vi "阈值设定.vi"() -> ()   [LabVIEW 2014]
uses:
  <vilib>/vision/Image Controls.llb/IMAQ Image.ctl
  <vilib>/Utility/error.llb/DialogType.ctl
  <vilib>/Utility/file.llb/Write To Spreadsheet File (I64).vi
  <vilib>/vision/NI_Vision_Development_Module.lvlib
panel:
  out "?":T1(plugin-control)
  in  "刷新按钮":bool
  in  "停止运算":bool
  in  "下一步":bool
  out "Histogram 3":dynamicdata(graph) caption="B直方图"
  out "Histogram 2":dynamicdata(graph) caption="A直方图"
  out "Histogram":dynamicdata(graph) caption="L直方图"
  in  "b颜色通道":cluster{i32, i32}(slide)={-21, 6} scale=-100.0..100.0
  in  "a颜色通道":cluster{i32, i32}(slide)={-21, -7} scale=-100.0..100.0
  in  "L颜色通道":cluster{i32, i32}(slide)={81, 99} scale=0.0..100.0
  out "lie":i32
  out "hang":i32
  out "颜色空间处理后的图，提取火焰":T1(plugin-control)
  in  "Image 4":T1
  out "B":u8[][](array[numeric])
  out "G":u8[][](array[numeric])
  out "R":u8[][](array[numeric])
  out "原图":T1(plugin-control)
  # "Lab颜色空间阈值选择"
  # "Lab颜色分割图像"
  # "滤波平滑图像"
  # "原图"
  # "阈\n值\n选\n择"
  # "火\n焰\n颜\n色\n直\n方\n图"
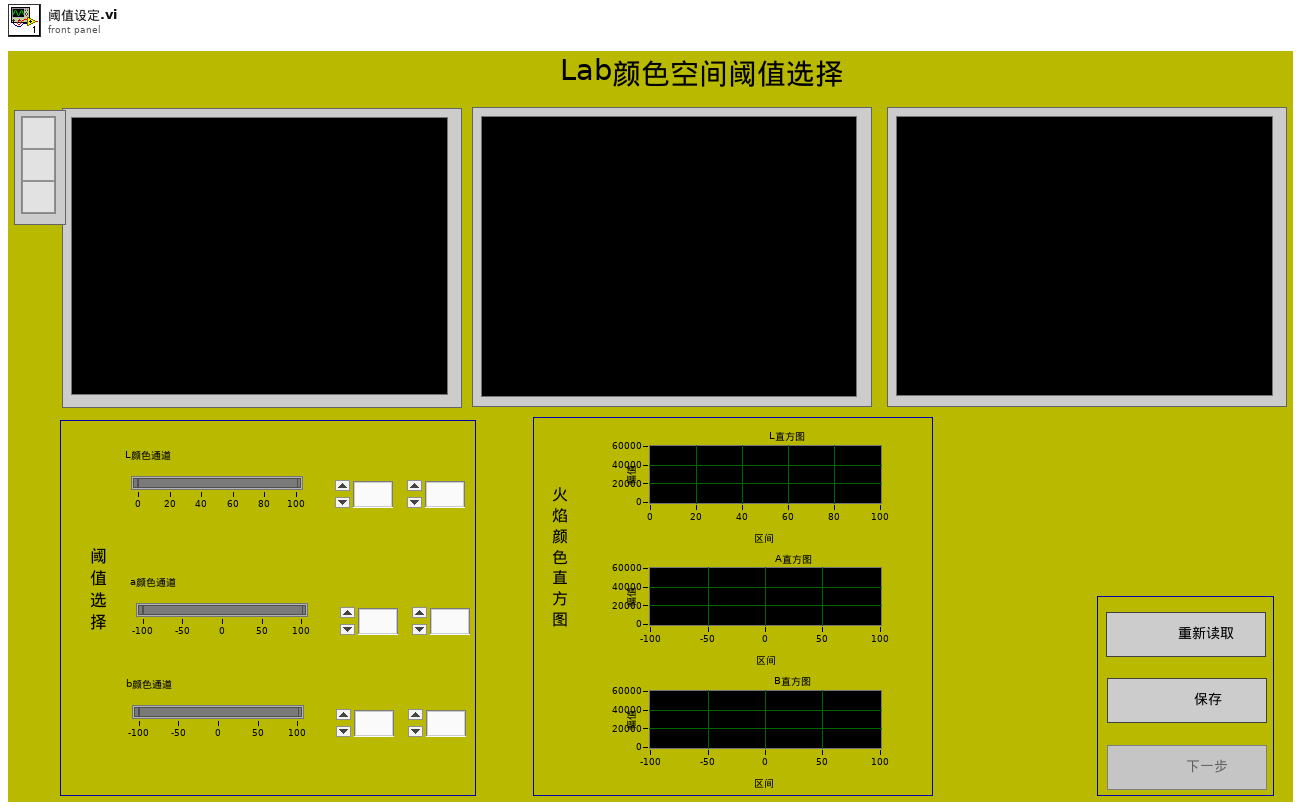
[diagram p1: front panel]
types:
  T1 = typedef "IMAQ Image.ctl" = refnum<image>
  T2 = enum8{"Enabled", "Disabled", "Disabled and Grayed Out"}
  T3 = enum32{"Invalid", "Standard", "Closed", "Hidden", "Minimized", "Maximized"}
  T4 = typedef "Image Type" = u32
  T5 = typedef "DialogType.ctl" = u16
  T6 = cluster{"Global Rectangle":i32[], "Contours":cluster{"Contour Type":u32, "ROI Type":u32, "Points":i32[]}[]}
  T7 = typedef "IMAQ Rectangle" = cluster{"Left":i32, "Top":i32, "Right":i32, "Bottom":i32, "Rotation":dbl}
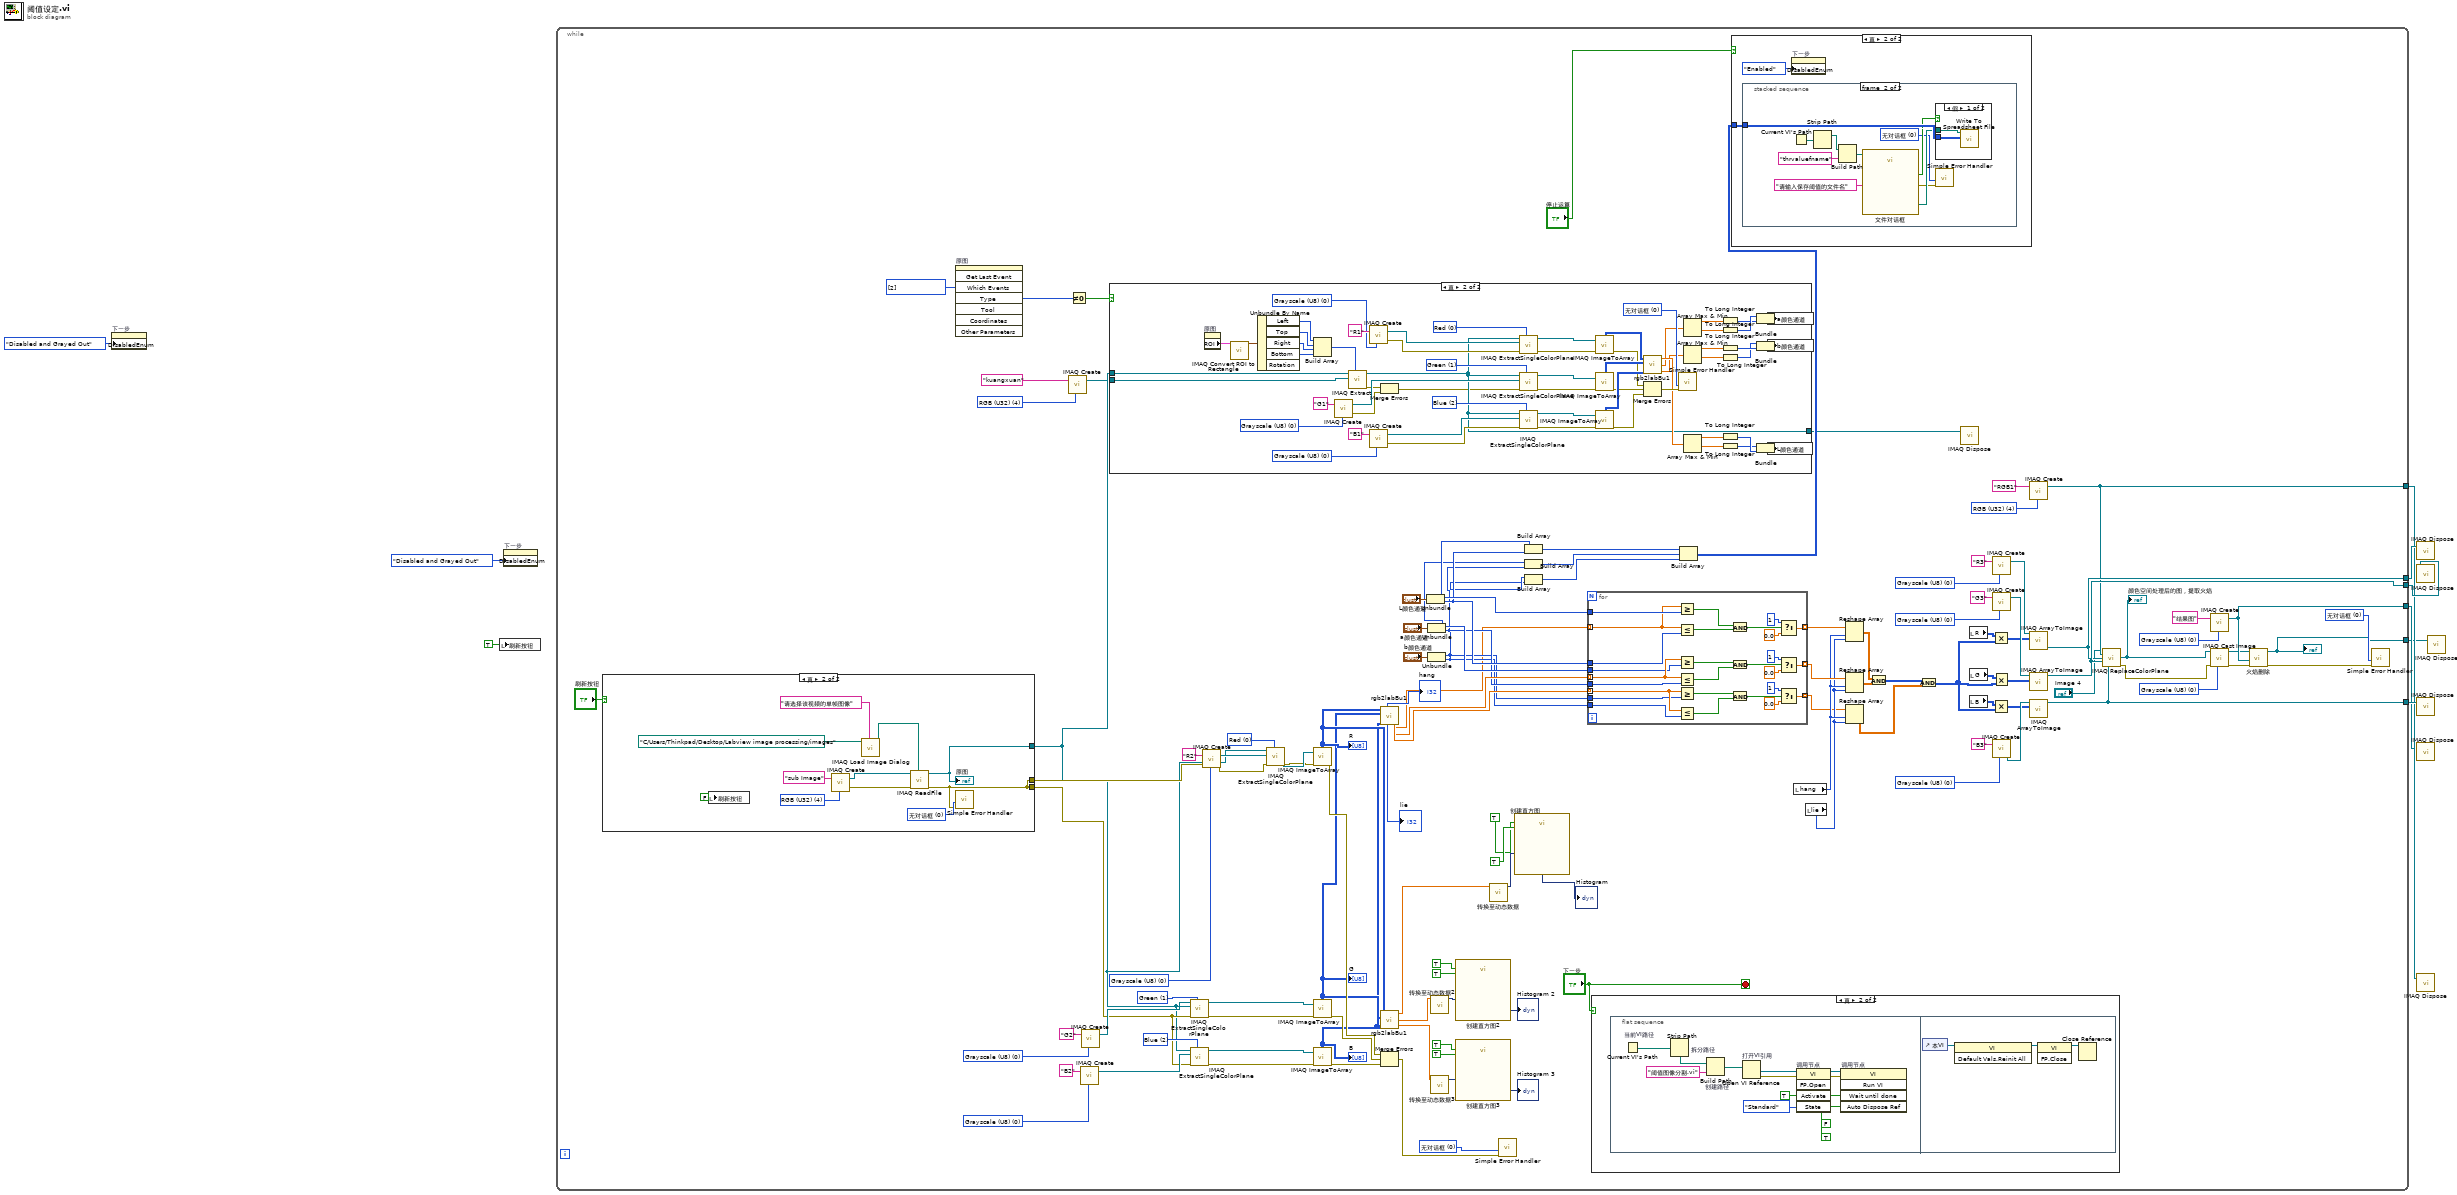
[diagram p0: block diagram]
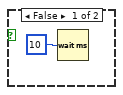
[diagram p2: hidden frame]
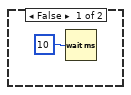
[diagram p3: hidden frame]
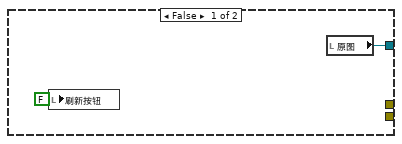
[diagram p4: hidden frame]
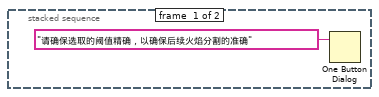
[diagram p6: hidden frame]
diagram:
  n1 = property on="下一步" class="Bool"("DisabledEnum"=T2."Disabled and Grayed Out" ("禁用")) -> ()  [unwired: 2 in, 2 out]
  n2 = local write "刷新按钮"(TRUE ("布尔")) -> ()
  n3 = property on="下一步" class="Bool"("DisabledEnum"=T2."Disabled and Grayed Out" ("禁用")) -> ()  [unwired: 2 in, 2 out]
  n4 = while {
    tunnel: [w125] -> w8
    tunnel: [w124] -> w7
    tunnel: [w123] -> w6
    tunnel: [w122] -> w5
    tunnel: [w121] -> w4
    tunnel: [w10] -> w1
    stop <- "下一步" stop-if-true
    w16 = T4 4 items=["Grayscale (U8)", "Grayscale (I16)", "Grayscale (SGL)", "Complex (CSG)", "RGB (U32)", "HSL (U32)", "RGB (U64)", "Grayscale (U16)"] ("Image Type")
    w15 = i32[] [2] items=["No  event", "Click event", "Draw event", "Move event", "Size event", "Scroll event", "Activate event", "Close event", "Double click event"] ("Events list (all)")
    w29 = T4 0 items=["Grayscale (U8)", "Grayscale (I16)", "Grayscale (SGL)", "Complex (CSG)", "RGB (U32)", "HSL (U32)", "RGB (U64)", "Grayscale (U16)"] ("Image Type")
    w27 = T4 0 items=["Grayscale (U8)", "Grayscale (I16)", "Grayscale (SGL)", "Complex (CSG)", "RGB (U32)", "HSL (U32)", "RGB (U64)", "Grayscale (U16)"] ("Image Type")
    w25 = T4 0 items=["Grayscale (U8)", "Grayscale (I16)", "Grayscale (SGL)", "Complex (CSG)", "RGB (U32)", "HSL (U32)", "RGB (U64)", "Grayscale (U16)"] ("Image Type")
    w56 = T5 0 items=["无对话框", "确定信息", "继续或停止信息", "确定信息＋警告", "继续/停止+警告"] ("type of dialog (OK msg:1)")
    w78 = T4 0 items=["Grayscale (U8)", "Grayscale (I16)", "Grayscale (SGL)", "Complex (CSG)", "RGB (U32)", "HSL (U32)", "RGB (U64)", "Grayscale (U16)"] ("Image Type")
    w79 = T4 4 items=["Grayscale (U8)", "Grayscale (I16)", "Grayscale (SGL)", "Complex (CSG)", "RGB (U32)", "HSL (U32)", "RGB (U64)", "Grayscale (U16)"] ("Image Type")
    w94 = T4 0 items=["Grayscale (U8)", "Grayscale (I16)", "Grayscale (SGL)", "Complex (CSG)", "RGB (U32)", "HSL (U32)", "RGB (U64)", "Grayscale (U16)"] ("Image Type")
    w100 = T4 0 items=["Grayscale (U8)", "Grayscale (I16)", "Grayscale (SGL)", "Complex (CSG)", "RGB (U32)", "HSL (U32)", "RGB (U64)", "Grayscale (U16)"] ("Image Type")
    w98 = T4 0 items=["Grayscale (U8)", "Grayscale (I16)", "Grayscale (SGL)", "Complex (CSG)", "RGB (U32)", "HSL (U32)", "RGB (U64)", "Grayscale (U16)"] ("Image Type")
    w103 = T4 0 items=["Grayscale (U8)", "Grayscale (I16)", "Grayscale (SGL)", "Complex (CSG)", "RGB (U32)", "HSL (U32)", "RGB (U64)", "Grayscale (U16)"] ("Image Type")
    w105 = T5 0 items=["无对话框", "确定信息", "继续或停止信息", "确定信息＋警告", "继续/停止+警告"] ("type of dialog (OK msg:1)")
    w114 = 2 items=["Red", "Green", "Blue", "Hue", "Saturation", "Luminance", "Value", "Intensity"] ("Color Plane")
    w115 = 1 items=["Red", "Green", "Blue", "Hue", "Saturation", "Luminance", "Value", "Intensity"] ("Color Plane")
    w116 = 0 items=["Red", "Green", "Blue", "Hue", "Saturation", "Luminance", "Value", "Intensity"] ("Color Plane")
    n5 = case shown="真" "刷新按钮" {
      tunnel: [_ w205] -> w20
      tunnel: [w203 w206] -> w19
      tunnel: [_ w205] -> w32
      frame False {
        n6 = local write "刷新按钮"(FALSE ("布尔")) -> ()
        n7 = local read "原图"() -> (w203:T1)
      }
      frame True {
        w210 = T5 0 items=["无对话框", "确定信息", "继续或停止信息", "确定信息＋警告", "继续/停止+警告"] ("type of dialog (OK msg:1)")
        w213 = T4 4 items=["Grayscale (U8)", "Grayscale (I16)", "Grayscale (SGL)", "Complex (CSG)", "RGB (U32)", "HSL (U32)", "RGB (U64)", "Grayscale (U16)"] ("Image Type")
        n8 = local write "刷新按钮"(FALSE ("布尔")) -> ()
        n9 = call "IMAQ Create"("Image Name"="sub Image", "Image Type"=w213) -> ("New Image"=w212:T1, "error out"=w211:errorcluster)  [unwired: 2 in, 1 out]
        n10 = call "IMAQ Load Image Dialog"("Prompt"="请选择该视频的单帧图像", "Start Path"=path "C:/Users/Thinkpad/Desktop/Labview image processing/images") -> ("Path"=w207:path)  [unwired: 7 in, 2 out]
        n11 = call "IMAQ ReadFile"("File Path"=w207, "error in (no error)"=w211, "Image"=w212) -> ("error out"=w205:errorcluster, "Image Out"=w206:T1)  [unwired: 4 in, 3 out]
        "原图" <- w206
        n12 = call <vilib>:"Simple Error Handler.vi"("type of dialog (OK msg:1)"=w210, "error in (no error)"=w205) -> ()  [unwired: 3 in, 5 out]
      }
    }
    n13 = invoke on="原图" class="ImageControl" method="Get Last Event"("Which Events"=w15) -> ("Type"=w14:i32)  [unwired: 7 in, 7 out]
    n14 = call "IMAQ Create"("Image Name"="kuangxuan", "Image Type"=w16) -> ("New Image"=w18:T1)  [unwired: 2 in, 2 out]
    n15 = Not Equal To 0?(x=w14) -> (x != 0?=w13:bool)
    n16 = call "IMAQ Create"("Image Name"="B2", "Image Type"=w29) -> ("New Image"=w24:T1)  [unwired: 2 in, 2 out]
    n17 = call "IMAQ Create"("Image Name"="G2", "Image Type"=w27) -> ("New Image"=w23:T1)  [unwired: 2 in, 2 out]
    n18 = case shown="真" w13 {
      tunnel: w18 -> [_ w148]
      tunnel: [_ w147] -> w12
      tunnel: w19 -> [_ w146]
      frame False {
        n19 = Wait (ms)(milliseconds to wait=u32 10) -> ()  [unwired: 1 out]
      }
      frame True {
        w178 = T5 0 items=["无对话框", "确定信息", "继续或停止信息", "确定信息＋警告", "继续/停止+警告"] ("type of dialog (OK msg:1)")
        w189 = 2 items=["Red", "Green", "Blue", "Hue", "Saturation", "Luminance", "Value", "Intensity"] ("Color Plane")
        w190 = 1 items=["Red", "Green", "Blue", "Hue", "Saturation", "Luminance", "Value", "Intensity"] ("Color Plane")
        w191 = 0 items=["Red", "Green", "Blue", "Hue", "Saturation", "Luminance", "Value", "Intensity"] ("Color Plane")
        w195 = T4 0 items=["Grayscale (U8)", "Grayscale (I16)", "Grayscale (SGL)", "Complex (CSG)", "RGB (U32)", "HSL (U32)", "RGB (U64)", "Grayscale (U16)"] ("Image Type")
        w197 = T4 0 items=["Grayscale (U8)", "Grayscale (I16)", "Grayscale (SGL)", "Complex (CSG)", "RGB (U32)", "HSL (U32)", "RGB (U64)", "Grayscale (U16)"] ("Image Type")
        w199 = T4 0 items=["Grayscale (U8)", "Grayscale (I16)", "Grayscale (SGL)", "Complex (CSG)", "RGB (U32)", "HSL (U32)", "RGB (U64)", "Grayscale (U16)"] ("Image Type")
        n20 = property on="原图" class="ImageControl"() -> ("ROI"=w149:T6)  [unwired: 2 in, 2 out]
        n21 = call "IMAQ Convert ROI to Rectangle"("ROI Descriptor"=w149) -> ("Rectangle"=w155:T7)  [unwired: 8 in, 1 out]
        n22 = Unbundle By Name(w155) -> ("Left"=w154:i32, "Top"=w153:i32, "Right"=w152:i32, "Bottom"=w151:i32)  [unwired: 1 out]
        n23 = Build Array(w154, w153, w152, w151) -> (w150:i32[])
        n24 = call "IMAQ Create"("Image Name"="G1", "Image Type"=w197) -> ("New Image"=w193:T1, "error out"=w144:errorcluster)  [unwired: 2 in, 1 out]
        n25 = call "IMAQ Extract"("Optional Rectangle"=w150, "Image Dst"=w148, "Image Src"=w146) -> ("error out"=w145:errorcluster, "Image Dst Out"=w147:T1)  [unwired: 7 in]
        n26 = call "IMAQ Create"("Image Name"="R1", "Image Type"=w199) -> ("New Image"=w194:T1, "error out"=w184:errorcluster)  [unwired: 2 in, 1 out]
        n27 = call "IMAQ Create"("Image Name"="B1", "Image Type"=w195) -> ("New Image"=w192:T1, "error out"=w201:errorcluster)  [unwired: 2 in, 1 out]
        n28 = Merge Errors(w145, w144) -> (w143:errorcluster)
        n29 = call "IMAQ ExtractSingleColorPlane"("Color Plane"=w191, "error in (no error)"=w184, "Image Dst"=w194, "Image Src"=w147) -> ("error out"=w183:errorcluster, "Image Dst Out"=w158:T1)  [unwired: 6 in]
        n30 = call "IMAQ ExtractSingleColorPlane"("Color Plane"=w190, "error in (no error)"=w143, "Image Dst"=w193, "Image Src"=w147) -> ("error out"=w185:errorcluster, "Image Dst Out"=w157:T1)  [unwired: 6 in]
        n31 = call "IMAQ ExtractSingleColorPlane"("Color Plane"=w189, "error in (no error)"=w201, "Image Dst"=w192, "Image Src"=w147) -> ("error out"=w182:errorcluster, "Image Dst Out"=w156:T1)  [unwired: 6 in]
        n32 = call "IMAQ ImageToArray"("error in (no error)"=w183, "Image"=w158) -> ("error out"=w181:errorcluster, "Image Pixels (U8)"=w188:u8[][])  [unwired: 2 in, 3 out]
        n33 = call "IMAQ ImageToArray"("error in (no error)"=w185, "Image"=w157) -> ("error out"=w180:errorcluster, "Image Pixels (U8)"=w187:u8[][])  [unwired: 2 in, 3 out]
        n34 = call "IMAQ ImageToArray"("error in (no error)"=w182, "Image"=w156) -> ("error out"=w179:errorcluster, "Image Pixels (U8)"=w186:u8[][])  [unwired: 2 in, 3 out]
        n35 = call "rgb2labBu1.vi"("R"=w188, "G"=w187, "B"=w186) -> ("LZ"=w171:dbl[], "aZ"=w160:dbl[], "bZ"=w159:dbl[])  [unwired: 1 in, 2 out]
        n36 = Merge Errors(w181, w180, w179) -> (w177:errorcluster)
        n37 = call <vilib>:"Simple Error Handler.vi"("type of dialog (OK msg:1)"=w178, "error in (no error)"=w177) -> ()  [unwired: 3 in, 5 out]
        n38 = Array Max & Min(array=w160) -> (max value=w166:dbl, min value=w167:dbl)  [unwired: 2 out]
        n39 = Array Max & Min(array=w159) -> (max value=w165:dbl, min value=w164:dbl)  [unwired: 2 out]
        n40 = Array Max & Min(array=w171) -> (max value=w176:dbl, min value=w175:dbl)  [unwired: 2 out]
        n41 = To Long Integer(number=w166) -> (32bit integer=w169:i32)
        n42 = To Long Integer(number=w167) -> (32bit integer=w170:i32)
        n43 = To Long Integer(number=w165) -> (32bit integer=w162:i32)
        n44 = To Long Integer(number=w164) -> (32bit integer=w161:i32)
        n45 = To Long Integer(number=w176) -> (32bit integer=w173:i32)
        n46 = To Long Integer(number=w175) -> (32bit integer=w172:i32)
        n47 = Bundle(w170, w169) -> (w168:cluster{i32, i32})  [unwired: 1 in]
        n48 = Bundle(w161, w162) -> (w163:cluster{i32, i32})  [unwired: 1 in]
        n49 = Bundle(w172, w173) -> (w174:cluster{i32, i32})  [unwired: 1 in]
        n50 = local write "a颜色通道"(w168) -> ()
        n51 = local write "b颜色通道"(w163) -> ()
        n52 = local write "L颜色通道"(w174) -> ()
      }
    }
    n53 = call "IMAQ ExtractSingleColorPlane"("Color Plane"=w115, "error in (no error)"=w20, "Image Dst"=w23, "Image Src"=w19) -> ("error out"=w111:errorcluster, "Image Dst Out"=w119:T1)  [unwired: 6 in]
    n54 = call "IMAQ ExtractSingleColorPlane"("Color Plane"=w114, "error in (no error)"=w20, "Image Dst"=w24, "Image Src"=w19) -> ("error out"=w109:errorcluster, "Image Dst Out"=w54:T1)  [unwired: 6 in]
    n55 = call "IMAQ Create"("Image Name"="R2", "Image Type"=w25, "error in (no error)"=w32) -> ("New Image"=w22:T1, "error out"=w21:errorcluster)  [unwired: 1 in, 1 out]
    n56 = call "IMAQ ExtractSingleColorPlane"("Color Plane"=w116, "error in (no error)"=w21, "Image Dst"=w22, "Image Src"=w19) -> ("error out"=w110:errorcluster, "Image Dst Out"=w120:T1)  [unwired: 6 in]
    n57 = call "IMAQ ImageToArray"("error in (no error)"=w110, "Image"=w120) -> ("error out"=w108:errorcluster, "Image Pixels (U8)"=w42:u8[][])  [unwired: 2 in, 3 out]
    "R" <- w42
    n58 = call "IMAQ ImageToArray"("error in (no error)"=w111, "Image"=w119) -> ("error out"=w107:errorcluster, "Image Pixels (U8)"=w41:u8[][])  [unwired: 2 in, 3 out]
    "G" <- w41
    n59 = call "IMAQ ImageToArray"("error in (no error)"=w109, "Image"=w54) -> ("error out"=w106:errorcluster, "Image Pixels (U8)"=w40:u8[][])  [unwired: 2 in, 3 out]
    "B" <- w40
    n60 = call "rgb2labBu1.vi"("R"=w42, "G"=w41, "B"=w40) -> ("hang"=→"hang":i32, "lie"=→"lie":i32, "LZ"=w53:dbl[], "aZ"=w117:dbl[], "bZ"=w118:dbl[])  [unwired: 1 in]
    n61 = call "rgb2labBu1.vi"("R"=w42, "G"=w41, "B"=w40) -> ("LZ"=w39:dbl[], "aZ"=w44:dbl[], "bZ"=w48:dbl[])  [unwired: 1 in, 2 out]
    n62 = Merge Errors(w108, w107, w106) -> (w104:errorcluster)
    n63 = Unbundle("L颜色通道") -> (w68:i32, w67:i32)
    n64 = Unbundle("a颜色通道") -> (w66:i32, w65:i32)
    n65 = Unbundle("b颜色通道") -> (w64:i32, w63:i32)
    n66 = call "转换至动态数据2"("Array"=w44) -> ("Dynamic Data Type"=w45:dynamicdata)  [unwired: 3 in]
    n67 = call "转换至动态数据3"("Array"=w48) -> ("Dynamic Data Type"=w49:dynamicdata)  [unwired: 3 in]
    n68 = call "创建直方图2"("Reset"=TRUE, "Enable"=TRUE, "Signal"=w45) -> ("Histogram"=→"Histogram 2":dynamicdata)  [unwired: 7 in, 1 out]
    n69 = call "创建直方图3"("Reset"=TRUE, "Enable"=TRUE, "Signal"=w49) -> ("Histogram"=→"Histogram 3":dynamicdata)  [unwired: 7 in, 1 out]
    n70 = call "转换至动态数据"("Array"=w39) -> ("Dynamic Data Type"=w43:dynamicdata)  [unwired: 3 in]
    n71 = call <vilib>:"Simple Error Handler.vi"("type of dialog (OK msg:1)"=w105, "error in (no error)"=w104) -> ()  [unwired: 3 in, 5 out]
    n72 = call "创建直方图"("Reset"=TRUE, "Enable"=TRUE, "Signal"=w43) -> ("Histogram"=→"Histogram":dynamicdata)  [unwired: 7 in, 1 out]
    n73 = Build Array(w68, w67) -> (w62:i32[])
    n74 = Build Array(w66, w65) -> (w61:i32[])
    n75 = Build Array(w64, w63) -> (w60:i32[])
    n76 = for {
      tunnel: w53 -> [w249] mode=indexing
      tunnel: w68 -> [w251]
      tunnel: w67 -> [w252]
      tunnel: [w253] -> w76 mode=indexing
      tunnel: w117 -> [w237] mode=indexing
      tunnel: w118 -> [w236] mode=indexing
      tunnel: w66 -> [w235]
      tunnel: w65 -> [w234]
      tunnel: w64 -> [w233]
      tunnel: w63 -> [w232]
      tunnel: [w231] -> w74 mode=indexing
      tunnel: [w230] -> w71 mode=indexing
      n77 = Greater Or Equal?(x=w249, y=w251) -> (x >= y?=w256:bool)
      n78 = Less Or Equal?(x=w249, y=w252) -> (x <= y?=w255:bool)
      n79 = Greater Or Equal?(x=w237, y=w235) -> (x >= y?=w247:bool)
      n80 = Less Or Equal?(x=w237, y=w234) -> (x <= y?=w246:bool)
      n81 = Greater Or Equal?(x=w236, y=w233) -> (x >= y?=w242:bool)
      n82 = Less Or Equal?(x=w236, y=w232) -> (x <= y?=w241:bool)
      n83 = And(x=w256, y=w255) -> (x .and. y?=w254:bool)
      n84 = And(x=w247, y=w246) -> (x .and. y?=w245:bool)
      n85 = And(x=w242, y=w241) -> (x .and. y?=w240:bool)
      n86 = Select(t=1, s=w254, f=0.0) -> (s? t:f=w253:dbl)
      n87 = Select(t=1, s=w245, f=0.0) -> (s? t:f=w231:dbl)
      n88 = Select(t=1, s=w240, f=0.0) -> (s? t:f=w230:dbl)
    }
    n89 = case shown="真" "下一步" {
      frame False {
        n90 = Wait (ms)(milliseconds to wait=u32 10 ("等待时间（毫秒）")) -> ()  [unwired: 1 out]
      }
      frame True {
        n91 = flat-sequence {
          frame #0 {
            n92 = Current VI's Path "当前VI路径"() -> (path=w135:path)
            n93 = Strip Path "拆分路径"(path=w135) -> (stripped path=w138:path)  [unwired: 1 out]
            n94 = Build Path "创建路径"(base path=w138, name or relative path="阈值图像分割.vi" ("名称或相对路径")) -> (appended path=w136:path)
            n95 = Open VI Reference "打开VI引用"(vi path=w136) -> (vi reference=w133:refnum<vi>, error out=w132:errorcluster)  [unwired: 5 in]
            n96 = invoke on="调用节点" class="VI" method="FP.Open"(reference=w133, error in=w132, "Activate"=TRUE ("激活？"), "State"=T3."Standard" ("状态")) -> (reference out=w131:refnum<vi>, error out=w130:errorcluster)  [unwired: 1 in, 3 out]
            n97 = invoke on="调用节点" class="VI" method="Run VI"(reference=w131, error in=w130, "Wait until done"=FALSE ("结束前等待"), "Auto Dispose Ref"=TRUE ("自动销毁引用")) -> ()  [unwired: 1 in, 5 out]
          }
          frame #1 {
            n98 = control-ref of="本VI"() -> (w141:refnum<vi>)
            n99 = invoke class="VI" method="Default Vals.Reinit All"(reference=w141) -> (reference out=w140:refnum<vi>)  [unwired: 2 in, 2 out]
            n100 = invoke class="VI" method="FP.Close"(reference=w140) -> (reference out=w139:refnum<vi>)  [unwired: 2 in, 2 out]
            n101 = Close Reference(reference=w139) -> ()  [unwired: 1 in, 1 out]
          }
        }
      }
    }
    n102 = Build Array(w62, w61, w60) -> (w59:i32[][])
    n103 = case shown="真" "停止运算" {
      tunnel: w59 -> [_ w216]
      frame False {
      }
      frame True {
        n104 = stacked-sequence {
          tunnel: w216 -> [_ w227]
          frame #0 {
            n105 = One Button Dialog(message="请确保选取的阈值精确，以确保后续火焰分割的准确" ("消息")) -> ()  [unwired: 1 in, 1 out]
          }
          frame #1 {
            w219 = T5 0 items=["无对话框", "确定信息", "继续或停止信息", "确定信息＋警告", "继续/停止+警告"] ("type of dialog (OK msg:1)")
            n106 = Current VI's Path() -> (path=w224:path)
            n107 = Strip Path(path=w224) -> (stripped path=w225:path)  [unwired: 1 out]
            n108 = Build Path(base path=w225, name or relative path="thrvaluefname" ("名称或相对路径")) -> (appended path=w223:path)
            n109 = call "文件对话框"("start path"=w223, "prompt"="请输入保存阈值的文件名") -> ("selected path"=w222:path, "cancelled"=w221:bool, "error out"=w220:errorcluster)  [unwired: 10 in, 1 out]
            n110 = case shown="假" w221 {
              tunnel: w227 -> [w229 _]
              tunnel: w222 -> [w228 _]
              frame False {
                n111 = call-poly <vilib>:"Write To Spreadsheet File.vi"("2D data"=w229, "file path (dialog if empty)"=w228) -> ()  [unwired: 6 in, 1 out]
              }
              frame True {
              }
            }
            n112 = call <vilib>:"Simple Error Handler.vi"("type of dialog (OK msg:1)"=w219, "error in (no error)"=w220) -> ()  [unwired: 3 in, 5 out]
          }
        }
        n113 = property on="下一步" class="Bool"("DisabledEnum"=T2."Enabled" ("禁用")) -> ()  [unwired: 2 in, 2 out]
      }
    }
    n114 = local read "hang"() -> (w73:i32)
    n115 = local read "lie"() -> (w72:i32)
    n116 = Reshape Array(w76, w73, w72) -> (w75:dbl[][])
    n117 = Reshape Array(w74, w73, w72) -> (w69:dbl[][])
    n118 = Reshape Array(w71, w73, w72) -> (w70:dbl[][])
    n119 = And(x=w75, y=w69) -> (x .and. y?=w92:i32[][])
    n120 = And(x=w92, y=w70) -> (x .and. y?=w85:i32[][])
    n121 = call "IMAQ Dispose"("Image"=w12) -> ()  [unwired: 5 in, 1 out]
    n122 = local read "R"() -> (w91:u8[][])
    n123 = local read "G"() -> (w90:u8[][])
    n124 = local read "B"() -> (w89:u8[][])
    n125 = call "IMAQ Create"("Image Name"="R3", "Image Type"=w103) -> ("New Image"=w101:T1)  [unwired: 2 in, 2 out]
    n126 = call "IMAQ Create"("Image Name"="G3", "Image Type"=w98) -> ("New Image"=w96:T1)  [unwired: 2 in, 2 out]
    n127 = Multiply(x=w91, y=w85) -> (x*y=w88:i32[][])
    n128 = Multiply(x=w89, y=w85) -> (x*y=w86:i32[][])
    n129 = call "IMAQ Create"("Image Name"="B3", "Image Type"=w100) -> ("New Image"=w95:T1)  [unwired: 2 in, 2 out]
    n130 = Multiply(x=w90, y=w85) -> (x*y=w87:i32[][])
    n131 = call "IMAQ Create"("Image Name"="RGB1", "Image Type"=w79) -> ("New Image"=w122:T1)  [unwired: 2 in, 2 out]
    n132 = call "IMAQ ArrayToImage"("Image Pixels (U8)"=w88, "Image"=w101) -> ("Image Out"=w123:T1)  [unwired: 8 in, 1 out]
    n133 = call "IMAQ ArrayToImage"("Image Pixels (U8)"=w87, "Image"=w96) -> ("Image Out"=w124:T1)  [unwired: 8 in, 1 out]
    n134 = call "IMAQ ArrayToImage"("Image Pixels (U8)"=w86, "Image"=w95) -> ("Image Out"=w125:T1)  [unwired: 8 in, 1 out]
    n135 = call "IMAQ ReplaceColorPlane"("Image Src"="Image 4", "Image Dst"=w122, "Red or Hue Plane"=w123, "Green or Sat Plane"=w124, "Blue or Luma or Val or Inten Plane"=w125) -> ("Image Dst Out"=w77:T1, "error out"=w58:errorcluster)  [unwired: 9 in]
    "颜色空间处理后的图，提取火焰" <- w77
    n136 = call "IMAQ Cast Image"("Image Type"=w78, "error in (no error)"=w58, "Image Src"=w77) -> ("error out"=w57:errorcluster, "Image Dst Out"=w81:T1)  [unwired: 7 in]
    n137 = call "IMAQ Create"("Image Name"="结果图", "Image Type"=w94) -> ("New Image"=w121:T1)  [unwired: 2 in, 2 out]
    n138 = call "火焰删除.vi"("error in (no error)"=w57, "Image dst"=w121, "Image source"=w81) -> ("error out"=w55:errorcluster, "Threshold Image"=w10:T1)  [unwired: 7 in]
    "?" <- w10
    n139 = call <vilib>:"Simple Error Handler.vi"("type of dialog (OK msg:1)"=w56, "error in (no error)"=w55) -> ()  [unwired: 3 in, 5 out]
  }
  n140 = call "IMAQ Dispose"("Image"=w6) -> ()  [unwired: 5 in, 1 out]
  n141 = call "IMAQ Dispose"("Image"=w7) -> ()  [unwired: 5 in, 1 out]
  n142 = call "IMAQ Dispose"("Image"=w8) -> ()  [unwired: 5 in, 1 out]
  n143 = call "IMAQ Dispose"("Image"=w4) -> ()  [unwired: 5 in, 1 out]
  n144 = call "IMAQ Dispose"("Image"=w5) -> ()  [unwired: 5 in, 1 out]
  n145 = call "IMAQ Dispose"("Image"=w1) -> ()  [unwired: 5 in, 1 out]
